vi "PLC_RE_Connect.vi"(7 "connect timeout ms":i32, 8 "error in (no error)":errorcluster, 9 "port (502)":u16, 10 "CID":string, 11 "Modbus Master in":refnum<class "Modbus Master.lvclass">) -> (0 "error out":errorcluster, 3 "Modbus Master out":refnum<class "Modbus Master.lvclass">)   [LabVIEW 2017]
uses:
  <vilib>/NI/Modbus Library/API/master/Modbus Master.lvclass
  <vilib>/NI/Modbus Library/API/Wrapper/Create TCP Master.vi
  <vilib>/NI/Modbus Library/API/Wrapper/API Main.lvlib
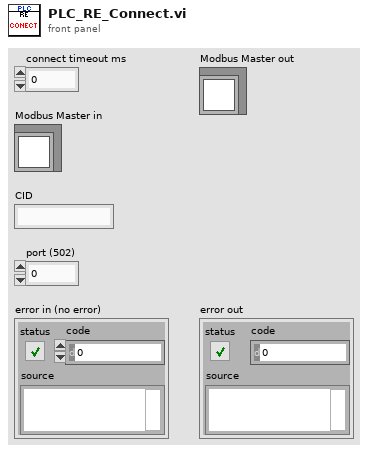
[diagram p1: front panel]
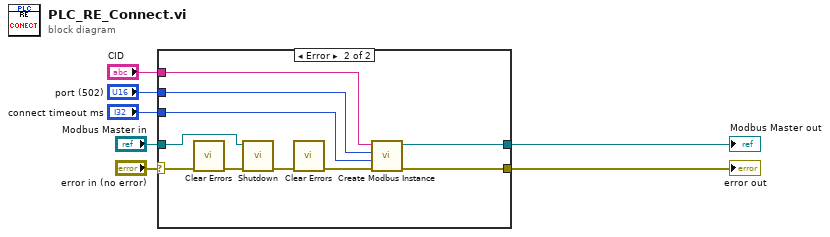
[diagram p0: block diagram]
diagram:
  n1 = case shown="Error" "error in (no error)" {
    selector: "error in (no error)" -> [w8 w14]
    tunnel: "Modbus Master in" -> [w9 w13]
    tunnel: [w9 w17] -> w7
    tunnel: [w8 w16] -> w6
    tunnel: "CID" -> [_ w10]
    tunnel: "port (502)" -> [_ w11]
    tunnel: "connect timeout ms" -> [_ w12]
    frame No Error {
    }
    frame Error {
      n2 = call <vilib>:"Clear Errors.vi"("error in (no error)"=w14) -> ("error out"=w15:errorcluster)  [unwired: 5 in, 1 out]
      n3 = call-dynamic "Shutdown.vi"("error in"=w15, "Modbus master in"=w13) -> ("error out"=w19:errorcluster)  [unwired: 9 in]
      n4 = call <vilib>:"Clear Errors.vi"("error in (no error)"=w19) -> ("error out"=w18:errorcluster)  [unwired: 5 in, 1 out]
      n5 = call-poly <vilib>:"Create Modbus Instance.vi"("error in"=w18, "connect timeout ms"=w12, "port (502)"=w11, "address"=w10) -> ("error out"=w16:errorcluster, "TCP master instance"=w17:refnum<class "Modbus Master.lvclass">)  [unwired: 6 in]
    }
  }
  "Modbus Master out" <- w7
  "error out" <- w6
